vi "Change IA settings.vi"(8 "error in (no error)":errorcluster, 11 "SysDef path in":path) -> (0 "error out":errorcluster, 3 "SysDef path out":path)   [LabVIEW 2018, in "Instrument Addon Common System Tests.lvclass"]
uses:
  Instrument Addon Common System Tests.lvclass
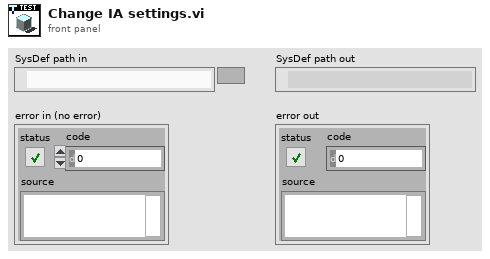
[diagram p1: front panel]
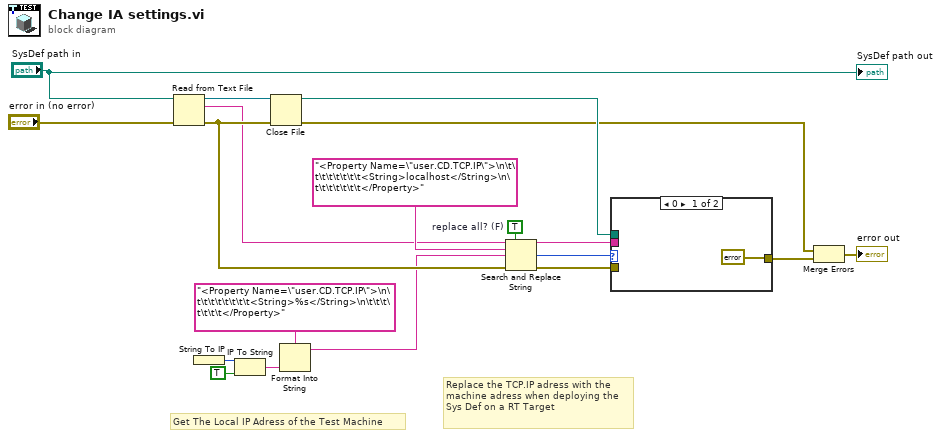
[diagram p0: block diagram]
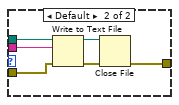
[diagram p2: hidden frame]
diagram:
  w9 = TRUE  # replace all? (F)
  # "Replace the TCP.IP adress with the machine adress when deploying the Sys Def on a RT Target"
  # "Get The Local IP Adress of the Test Machine"
  n1 = Read from Text File(file (use dialog)="SysDef path in", error in="error in (no error)") -> (refnum out=w7:refnum<file>, text=w12:string, error out=w15:errorcluster)  [unwired: 2 in, 1 out]
  n2 = String To IP() -> (0:w4:u32)  [unwired: 1 in]
  n3 = IP To String(1:TRUE ("dot notation? (F)"), 2:w4) -> (0:w3:string)
  n4 = Close File(refnum=w7, error in=w15) -> (path=w18:path, error out=w17:errorcluster)
  n5 = Format Into String(format string="<Property Name=\"user.CD.TCP.IP\">\n\t\t\t\t\t\t\t\t<String>%s</String>\n\t\t\t\t\t\t\t</Property>" ("search string"), w3) -> (resulting string=w5:string)  [unwired: 2 in, 1 out]
  n6 = Search and Replace String(replace all?=w9, input string=w12, search string="<Property Name=\"user.CD.TCP.IP\">\n\t\t\t\t\t\t\t\t<String>localhost</String>\n\t\t\t\t\t\t\t</Property>", replace string=w5, error in=w15) -> (result string=w10:string, number of replacements=w19:i32, error out=w11:errorcluster)  [unwired: 3 in, 1 out]
  n7 = case shown="0" w19 {
    tunnel: w10 -> [_ w24]
    tunnel: w11 -> [_ w23]
    tunnel: [errorcluster {"status"=FALSE, "code"=0, "source"=""} ("error out") w22] -> w14
    tunnel: w18 -> [_ w21]
    frame 0 {
    }
    frame Default {
      n8 = Write to Text File(file (use dialog)=w21, text=w24, error in=w23) -> (refnum out=w25:refnum<file>, error out=w26:errorcluster)  [unwired: 1 in, 1 out]
      n9 = Close File(refnum=w25, error in=w26) -> (error out=w22:errorcluster)  [unwired: 1 out]
    }
  }
  n10 = Merge Errors(w17, w14) -> (→"error out":errorcluster)
  "SysDef path out" <- "SysDef path in"
